vi "Update display target.vi"(8 "error in (no error)":errorcluster, 11 "StageSPIM in":refnum<class "StageSPIM.lvclass">) -> (0 "error out":errorcluster, 3 "StageSPIM out":refnum<class "StageSPIM.lvclass">)   [LabVIEW 2012, in "StageSPIM.lvclass"]
uses:
  StageSPIM.lvclass
  StageSPIM.lvclass/StageSPIM.ctl
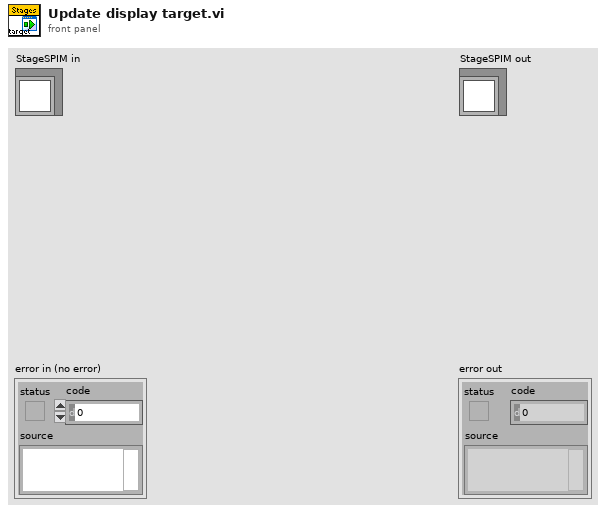
[diagram p1: front panel]
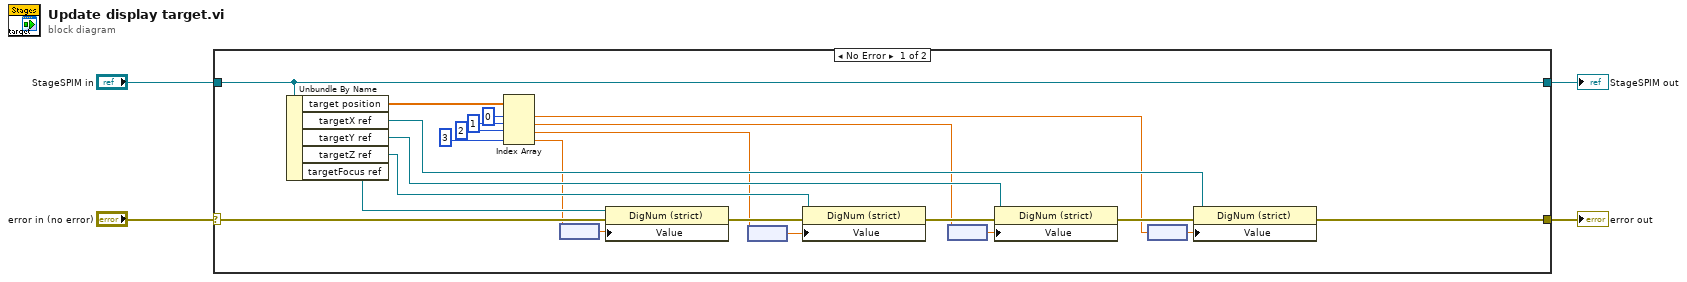
[diagram p0: block diagram]
diagram:
  n1 = case shown="No Error" "error in (no error)" {
    selector: "error in (no error)" -> [w13 w29]
    tunnel: [w9 w29] -> w3
    tunnel: [w15 w28] -> w1
    tunnel: "StageSPIM in" -> [w15 w28]
    frame No Error {
      n2 = Unbundle By Name(w15) -> ("target position"=w27:dbl[], "targetX ref"=w21:refnum<vi>, "targetY ref"=w14:refnum<vi>, "targetZ ref"=w22:refnum<vi>, "targetFocus ref"=w10:refnum<vi>)
      n3 = Index Array(array=w27, index #1=0 ("index"), index #2=1 ("index"), index #3=2 ("index"), index #4=3 ("index")) -> (element #1=w8:dbl, element #2=w7:dbl, element #3=w6:dbl, element #4=w5:dbl)
      n4 = node(w5) -> (w11:dbl[unit])
      n5 = property class="DigNum (strict)"(reference=w10, error in=w13, "Value"=w11) -> (error out=w12:errorcluster)  [unwired: 1 out]
      n6 = node(w6) -> (w18:dbl[unit])
      n7 = property class="DigNum (strict)"(reference=w22, error in=w12, "Value"=w18) -> (error out=w20:errorcluster)  [unwired: 1 out]
      n8 = node(w7) -> (w17:dbl[unit])
      n9 = property class="DigNum (strict)"(reference=w14, error in=w20, "Value"=w17) -> (error out=w19:errorcluster)  [unwired: 1 out]
      n10 = node(w8) -> (w16:dbl[unit])
      n11 = property class="DigNum (strict)"(reference=w21, error in=w19, "Value"=w16) -> (error out=w9:errorcluster)  [unwired: 1 out]
    }
    frame Error {
    }
  }
  "error out" <- w3
  "StageSPIM out" <- w1
